vi "Demultiplexer_Laser80Simple160.vi"() -> ()   [LabVIEW 2012]
uses:
  <vilib>/Platform/TimedLoop/XDataNode/timing_clust.ctl
  <vilib>/Platform/TimedLoop/XDataNode/nitl_modes.ctl
  <vilib>/Platform/TimedLoop/XDataNode/wakeup.ctl
  <vilib>/rvi/Emulation/niFpgaSctlEmulationRegisterWithScheduler.vi
  <vilib>/rvi/eio/common/nirviEmuTemplateMethod_errors.vi
  <vilib>/rvi/Emulation/niFpgaSctlEmulationScheduler.vi
  <vilib>/rvi/FIFO/Fifo_Resource/nirvififoEmulationSetSize.vi
  <vilib>/rvi/DataTransferAndStorage/Container/Common/niFpgaContainerGetUniqueNameForEmu.vi
  <vilib>/rvi/errors/niFpgaSetErrorForExecOnDevCompSimple.vi
  <vilib>/rvi/eio/common/nirviEmuReportErrorAndStop.vi
  <vilib>/rvi/Emulation/niFpgaSctlEmulationFifoFullMgr.vi
  <vilib>/rvi/Emulation/niFpgaSctlEmulationResourceMgr.vi
  <vilib>/rvi/interface/RandomDataEmulation/nirviRandomDataFPGAFIFO.vi
  <vilib>/rvi/interface/RandomDataEmulation/niFpgaRandomDataHandleErrors.vi
  <vilib>/rvi/Emulation/niFpgaSctlEmulationGlobalWrite.vi
  <vilib>/Platform/TimedLoop/XDataNode/XDataNode.xnode
  <vilib>/eio/EIONode/EIONode.xnode
  <vilib>/rvi/DataTransferAndStorage/Container/XNode/niFpgaContainer.xnode
  <vilib>/rvi/FIFO/Fifo_Resource/nirvififoEmulationClear.vi
  <vilib>/rvi/FIFO/Fifo_Resource/nirvififoEmulationWrite.vi
  <vilib>/rvi/FIFO/Fifo_Resource/nirvififoEmulationRead.vi
  <vilib>/rvi/interface/RandomDataEmulation/nirviRandomDataFpgaReadWriteTemplate.vi
  <vilib>/Platform/TimedLoop/XDataNode/XDNodeRunTimeDep.lvlib
panel:
  out "Laser pulse count A1":u16
  out "ToHost FIFO Overflow A2Ch2":bool
  out "ToHost FIFO Overflow A2Ch1":bool
  out "ToHost FIFO Overflow A1Ch2":bool
  in  "Samples per pixel Acq A2":u16=10000 caption="Samples per pixel Acq"
  in  "Samples per pixel Acq A1":u16=10000 caption="Samples per pixel Acq"
  in  "Requested pixels A2":u32=100000 caption="Requested pixels"
  in  "Samples per pixel A2":u16=10000 caption="Samples per pixel"
  out "ToHost FIFO Overflow A1Ch1":bool
  out "Acquiring":bool
  in  "Wait for trigger":bool
  in  "Acquire continuously":bool=TRUE
  in  "Requested pixels A1":u32=100000 caption="Requested pixels"
  in  "Clear Interloop FIFO":bool
  out "Interloop FIFO overflow":bool
  in  "Samples per pixel A1":u16=10000 caption="Samples per pixel"
  in  "Acquire":bool
  out "Interloop FIFO timeout":bool
  in  "Commit":bool
  out "Xpoint_Switch_Ready":bool
  in  "Xpoint_Switch_Write":bool
  in  "Clock Source":u8(ring)=3 items=["Tristate"=0, "Sync Clock (PXIe only)"=2, "Adapter Module Onboard Clock"=3, "Strobe from Crosspoint Switch"=4, "Strobe Bypass"=5]
  in  "Onboard_Clock_Write":bool
  in  "Onboard_Clock_Write_Data":u16
  out "Onboard_Clock_Ready":bool
  in  "Acq_Reset":bool
  # "6587 IO module configuration"
  # "Demultiplexer - Laser 80MHzSimple160MHz"
  # "Acquisition control"
  # "Area 1"
  # "Area 2"
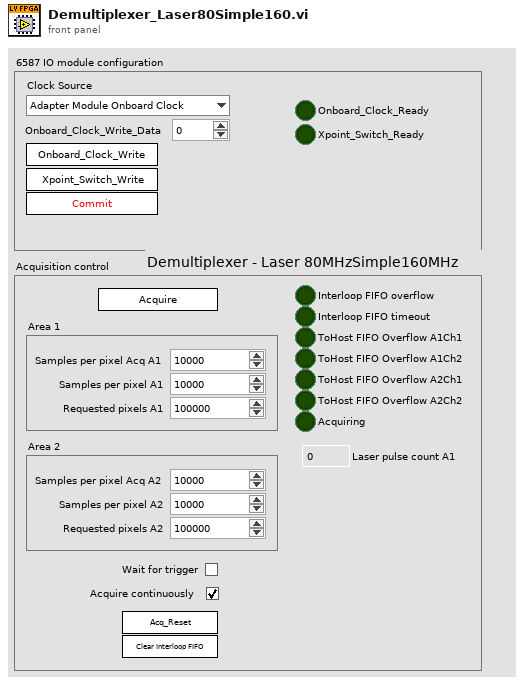
[diagram p1: front panel]
types:
  T1 = typedef "XDNodeRunTimeDep.lvlib/timing_clust.ctl" = cluster{"Expected End [f-1]":u64, "Actual End [f-1]":u64, "Finished Late? [f-1]":bool, "Expected End [i-1]":u64, "Actual End [i-1]":u64, "Finished Late? [i-1]":bool, "Expected Start [i]":u64, "Actual Start [i]":u64, "Expected Start [f]":u64, "Actual Start [f]":u64, "Source Name":string, "Structure Name":string, "Period":i64, "Deadline":i64, "Offset":i64, "Start":i64, "Priority":i32, "Timeout":i32, "Mode":T2, "Wakeup Reason":T3, "Error":errorcluster, "Source Type":string, "Secondary Source Type":string, "Global End Time":u64, "Global Start Time":u64, "Frame Duration":u64, "Iteration Duration":u64, "Assigned CPU":i32, "I/O Scan Engine Mode":u32}
  T2 = typedef "XDNodeRunTimeDep.lvlib/nitl_modes.ctl" = enum32{"No Change", "Process missed periods, maintain original phase", "Discard missed periods, maintain original phase", "Process missed periods, ignore original phase", "Discard missed periods, ignore original phase"}
  T3 = typedef "XDNodeRunTimeDep.lvlib/wakeup.ctl" = enum32{"Normal", "Aborted", "Asynchronous wakeup", "Timing source error", "Timed loop error", "Timeout"}
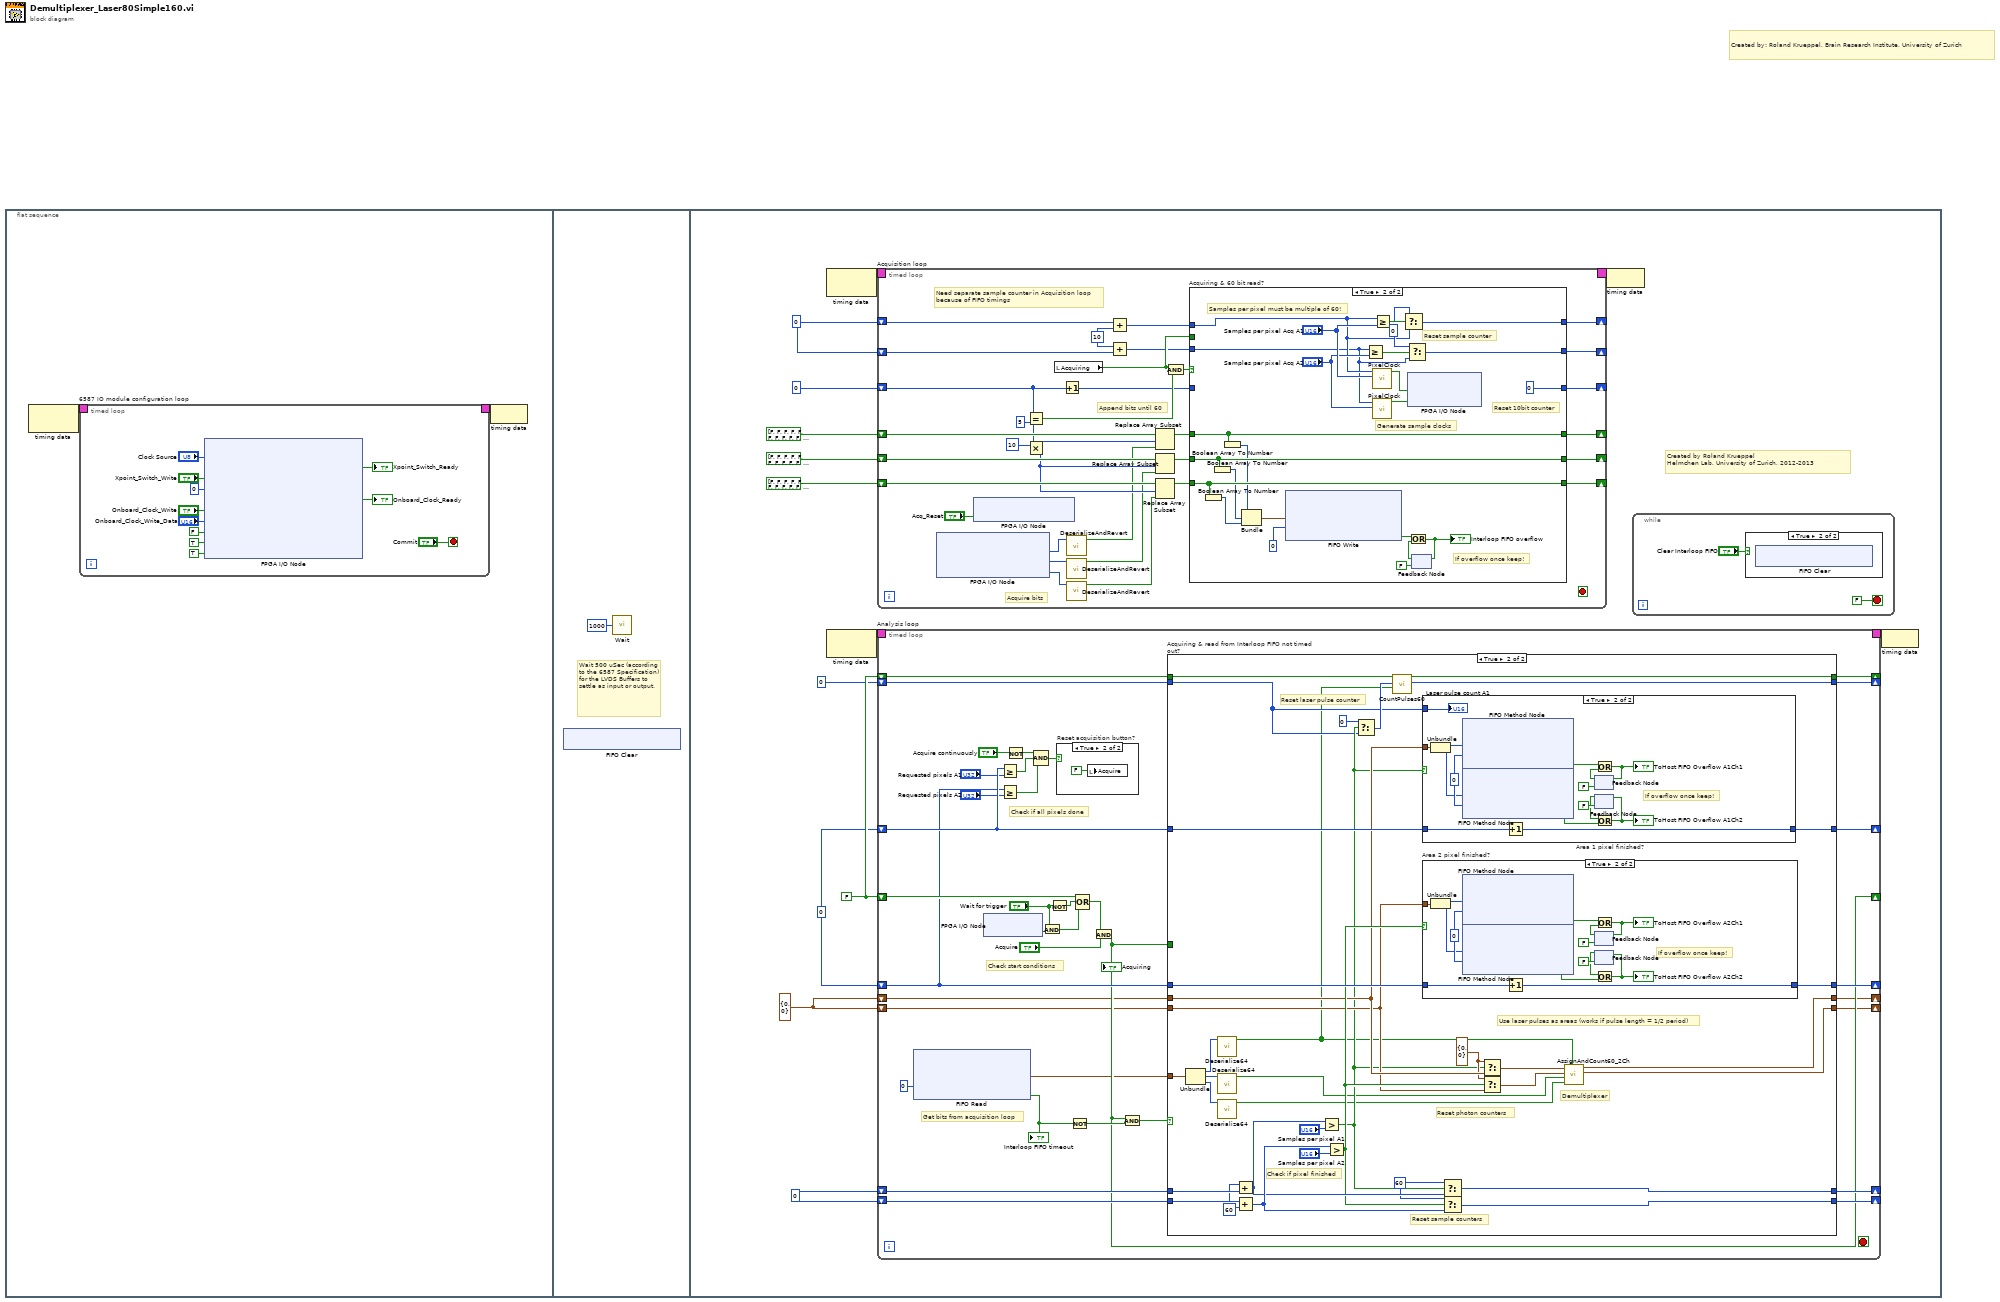
[diagram p0: block diagram]
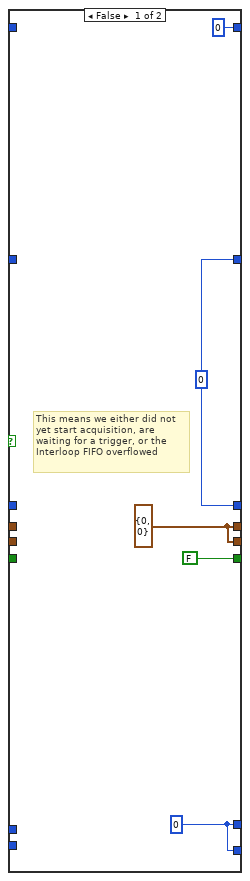
[diagram p5: hidden frame]
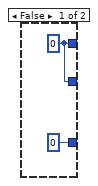
[diagram p9: hidden frame]
diagram:
  # "Created by: Roland Krueppel, Brain Research Institute, University of Zurich"
  n1 = flat-sequence {
    frame #0 {
      n2 = node-c288() -> (w2:T1)  [unwired: 1 in]
      n3 = timed-loop "6587 IO module configuration loop" {
        timing: w2 -> [_]
        timing-out: [_] -> w1
        stop <- "Commit" stop-if-true
        n4 = xnode "FPGA I/O Node"("IO Module\\Acq_IO_Clock_Source"="Clock Source", "IO Module\\Xpoint_Switch_Write"="Xpoint_Switch_Write", "IO Module\\LVDS_Data_Dir"=u16 0 ("IO Module\\LVDS_Data_Dir"), "IO Module\\Onboard_Clock_Write"="Onboard_Clock_Write", "IO Module\\Onboard_Clock_Write_Data"="Onboard_Clock_Write_Data", "IO Module\\SE_PFI0_WE"=FALSE ("IO Module\\SE_PFI0_WE"), "IO Module\\SE_PFI1_WE"=TRUE ("IO Module\\SE_PFI1_WE"), "IO Module\\SE_PFI2_WE"=TRUE ("IO Module\\SE_PFI2_WE")) -> ("IO Module\\Xpoint_Switch_Ready"=→"Xpoint_Switch_Ready":bool, "IO Module\\Onboard_Clock_Ready"=→"Onboard_Clock_Ready":bool)  [unwired: 10 in, 10 out]
      }
      n5 = node-c288(w1) -> ()
    }
    frame #1 {
      # "Wait 500 uSec (according to the 6587 Specification) for the LVDS Buffers to settle as input or output."
      n6 = xnode "FIFO Clear"() -> ()  [unwired: 1 in, 1 out]
      n7 = call "Wait"("Count(uSec)"=u32 1000) -> ()  [unwired: 1 out]
    }
    frame #2 {
      w21 = cluster{u16, u16} {0, 0} ("output cluster")
      w22 = u16 0
      w20 = u32 0 ("Cycle counter out")
      w23 = u16 0
      w24 = FALSE ("Last laser bit out")
      # "Created by Roland Krueppel\nHelmchen Lab, University of Zurich, 2012-2013"
      n8 = node-c288() -> (w32:T1)  [unwired: 1 in]
      n9 = node-c288() -> (w30:T1)  [unwired: 1 in]
      n10 = timed-loop "Acquisition loop" {
        timing: w32 -> [_]
        timing-out: [_] -> w31
        shift-right: [w195] -> _
        shift-left: bool[] [FALSE, FALSE, FALSE, FALSE, FALSE, FALSE, FALSE, FALSE, FALSE, FALSE, FALSE, FALSE, FALSE, FALSE, FALSE, FALSE, FALSE, FALSE, FALSE, FALSE, FALSE, FALSE, FALSE, FALSE, FALSE, FALSE, FALSE, FALSE, FALSE, FALSE, FALSE, FALSE, FALSE, FALSE, FALSE, FALSE, FALSE, FALSE, FALSE, FALSE, FALSE, FALSE, FALSE, FALSE, FALSE, FALSE, FALSE, FALSE, FALSE, FALSE, FALSE, FALSE, FALSE, FALSE, FALSE, FALSE, FALSE, FALSE, FALSE, FALSE, FALSE, FALSE, FALSE, FALSE] ("Boolean array") -> [w203]
        shift-right: [w194] -> _
        shift-left: bool[] [FALSE, FALSE, FALSE, FALSE, FALSE, FALSE, FALSE, FALSE, FALSE, FALSE, FALSE, FALSE, FALSE, FALSE, FALSE, FALSE, FALSE, FALSE, FALSE, FALSE, FALSE, FALSE, FALSE, FALSE, FALSE, FALSE, FALSE, FALSE, FALSE, FALSE, FALSE, FALSE, FALSE, FALSE, FALSE, FALSE, FALSE, FALSE, FALSE, FALSE, FALSE, FALSE, FALSE, FALSE, FALSE, FALSE, FALSE, FALSE, FALSE, FALSE, FALSE, FALSE, FALSE, FALSE, FALSE, FALSE, FALSE, FALSE, FALSE, FALSE, FALSE, FALSE, FALSE, FALSE] ("Boolean array") -> [w202]
        shift-right: [w193] -> _
        shift-left: 0 -> [w192]
        shift-right: [w188] -> _
        shift-left: bool[] [FALSE, FALSE, FALSE, FALSE, FALSE, FALSE, FALSE, FALSE, FALSE, FALSE, FALSE, FALSE, FALSE, FALSE, FALSE, FALSE, FALSE, FALSE, FALSE, FALSE, FALSE, FALSE, FALSE, FALSE, FALSE, FALSE, FALSE, FALSE, FALSE, FALSE, FALSE, FALSE, FALSE, FALSE, FALSE, FALSE, FALSE, FALSE, FALSE, FALSE, FALSE, FALSE, FALSE, FALSE, FALSE, FALSE, FALSE, FALSE, FALSE, FALSE, FALSE, FALSE, FALSE, FALSE, FALSE, FALSE, FALSE, FALSE, FALSE, FALSE, FALSE, FALSE, FALSE, FALSE] ("Boolean array") -> [w191]
        shift-right: [w187] -> _
        shift-left: w22 -> [w177]
        shift-right: [w186] -> _
        shift-left: w22 -> [w175]
        stop <- _ stop-if-true
        w173 = u16 10 ("y")
        # "Need separate sample counter in Acquisition loop\nbecause of FIFO timings"
        # "Append bits until 60"
        # "Acquire bits"
        n11 = xnode "FPGA I/O Node"() -> ("IO Module\\LVDS_Ch0_Rd"=w183:u16, "IO Module\\LVDS_Ch1_Rd"=w181:u16, "IO Module\\LVDS_Ch2_Rd"=w179:u16)  [unwired: 3 in, 3 out]
        n12 = xnode "FPGA I/O Node"("IO Module\\Acq_Reset"="Acq_Reset") -> ()  [unwired: 1 in, 1 out]
        n13 = Equal?(x=w192, y=5) -> (x = y?=w199:bool)
        n14 = Multiply(x=10 ("y"), y=w192) -> (x*y=w190:i32)
        n15 = local read "Acquiring"() -> (w185:bool)
        n16 = Increment(x=w192) -> (x+1=w184:i32)
        n17 = call "DeserializeAndRevert.vi"("U16 input"=w183) -> ("10bit output"=w182:bool[])  [unwired: 10 in]
        n18 = call "DeserializeAndRevert.vi"("U16 input"=w181) -> ("10bit output"=w180:bool[])  [unwired: 10 in]
        n19 = call "DeserializeAndRevert.vi"("U16 input"=w179) -> ("10bit output"=w178:bool[])  [unwired: 10 in]
        n20 = Add(x=w177, y=w173) -> (x+y=w176:u16)
        n21 = Add(x=w173, y=w175) -> (x+y=w174:u16)
        n22 = Replace Array Subset(array=w203, new element=w182, index=w190) -> (w197:bool[])
        n23 = Replace Array Subset(array=w202, new element=w180, index=w190) -> (w196:bool[])
        n24 = Replace Array Subset(array=w191, new element=w178, index=w190) -> (w189:bool[])
        n25 = And(x=w185, y=w199) -> (x .and. y?=w198:bool)
        n26 = case "Acquiring & 60 bit read?" shown="True" w198 {
          tunnel: w197 -> [w214 w240]
          tunnel: w196 -> [w213 w242]
          tunnel: [w214 w240] -> w195
          tunnel: [w213 w242] -> w194
          tunnel: [w205 0] -> w193
          tunnel: w184 -> [w206 _]
          tunnel: w189 -> [w212 w241]
          tunnel: [w212 w241] -> w188
          tunnel: w176 -> [w210 w225]
          tunnel: [w207 w238] -> w187
          tunnel: w174 -> [w209 w224]
          tunnel: [w208 w233] -> w186
          tunnel: w185 -> [w211 _]
          frame False {
            n27 = case "Acquiring?" shown="True" w211 {
              tunnel: w210 -> [_ w219]
              tunnel: w209 -> [_ w218]
              tunnel: [w216 w219] -> w207
              tunnel: [w216 w218] -> w208
              tunnel: w206 -> [_ w217]
              tunnel: [0 w217] -> w205
              frame False {
                w216 = u16 0
              }
              frame True {
              }
            }
          }
          frame True {
            w234 = u16 0 ("t")
            # "Reset 10bit counter"
            # "Samples per pixel must be multiple of 60!"
            # "Reset sample counter"
            # "If overflow once keep!"
            # "Generate sample clocks"
            n28 = Boolean Array To Number(Boolean array=w241) -> (number=w228:u64)
            n29 = Boolean Array To Number(Boolean array=w242) -> (number=w229:u64)
            n30 = Boolean Array To Number(Boolean array=w240) -> (number=w230:u64)
            n31 = Bundle(w230, w229, w228) -> (w227:cluster{u64, u64, u64})  [unwired: 1 in]
            n32 = xnode ("FIFO Write")("Element"=w227, "Timeout"=0) -> ("Timed Out?"=w223:bool)  [unwired: 1 in, 1 out]
            n33 = Greater Or Equal?(x=w224, y="Samples per pixel Acq A2") -> (x >= y?=w235:bool)
            n34 = call "PixelClock.vi"("Samples per pixel"="Samples per pixel Acq A1", "Sample counter"=w225) -> ("Pixel clock"=w236:bool)  [unwired: 9 in]
            n35 = call "PixelClock.vi"("Samples per pixel"="Samples per pixel Acq A2", "Sample counter"=w224) -> ("Pixel clock"=w231:bool)  [unwired: 9 in]
            n36 = Greater Or Equal?(x=w225, y="Samples per pixel Acq A1") -> (x >= y?=w239:bool)
            n37 = Select(t=w234, s=w239, f=w225) -> (s? t:f=w238:u16)
            n38 = Select(t=w234, s=w235, f=w224) -> (s? t:f=w233:u16)
            n39 = xnode "FPGA I/O Node"("Pixel clock A1"=w236, "Pixel clock A2"=w231) -> ()  [unwired: 2 in, 2 out]
            n40 = feedback #1(FALSE) -> (w221:bool)
            n41 = Or(x=w223, y=w221) -> (x .or. y?=w222:bool)
            "Interloop FIFO overflow" <- w222
            n42 = feedback-in #1(w222) -> ()
          }
        }
      }
      n43 = timed-loop "Analysis loop" {
        timing: w30 -> [_]
        timing-out: [_] -> w29
        shift-right: [w70] -> _
        shift-left: w24 -> [w69]
        shift-right: [w48] -> _
        shift-left: w23 -> [w68]
        shift-right: [w46] -> _
        shift-left: w20 -> [w67]
        shift-right: [w44] -> _
        shift-left: w24 -> [w56]
        shift-right: [w47] -> _
        shift-left: w23 -> [w54]
        shift-right: [w45] -> _
        shift-left: w20 -> [w52]
        shift-right: [w39] -> _
        shift-left: w21 -> [w41]
        shift-right: [w38] -> _
        shift-left: w21 -> [w40]
        shift-right: [w37] -> _
        shift-left: u16 0 ("New pulse count") -> [w36]
        stop <- _ stop-if-true
        # "Get bits from acquisition loop"
        # "Check start conditions"
        # "Check if all pixels done"
        n44 = xnode ("FIFO Read")("Timeout"=0) -> ("Element"=w35:cluster{"Laser":u64, "Ch0":u64, "Ch1":u64}, "Timed Out?"=w42:bool)  [unwired: 1 in, 1 out]
        "Interloop FIFO timeout" <- w42
        n45 = xnode "FPGA I/O Node"() -> ("TriggerIn"=w62:bool)  [unwired: 1 in, 1 out]
        n46 = Greater Or Equal?(x=w67, y="Requested pixels A1") -> (x >= y?=w50:bool)
        n47 = Greater Or Equal?(x=w52, y="Requested pixels A2") -> (x >= y?=w49:bool)
        n48 = Not(x="Acquire continuously") -> (.not. x?=w51:bool)
        n49 = Compound Arithmetic op=AND(w51, w50, w49) -> (w64:bool)
        n50 = And(x="Wait for trigger", y=w62) -> (x .and. y?=w59:bool)
        n51 = Not(x="Wait for trigger") -> (.not. x?=w60:bool)
        n52 = case "Reset acquisition button?" shown="True" w64 {
          frame False {
          }
          frame True {
            n53 = local write "Acquire"(FALSE ("Acquire")) -> ()
          }
        }
        n54 = Not(x=w42) -> (.not. x?=w57:bool)
        n55 = Compound Arithmetic op=OR(w56, w60, w59) -> (w58:bool)
        n56 = And(x=w58, y="Acquire") -> (x .and. y?=w44:bool)
        "Acquiring" <- w44
        n57 = And(x=w44, y=w57) -> (x .and. y?=w55:bool)
        n58 = case "Acquiring & read from Interloop FIFO not timed out?" shown="True" w55 {
          tunnel: w41 -> [w87 w122]
          tunnel: [w83 w102] -> w70
          tunnel: w69 -> [w84 w111]
          tunnel: w68 -> [w86 w137]
          tunnel: w67 -> [w85 w133]
          tunnel: w44 -> [w88 _]
          tunnel: w54 -> [w77 w135]
          tunnel: w52 -> [w80 w132]
          tunnel: [w78 w125] -> w48
          tunnel: [w76 w127] -> w47
          tunnel: [w82 w117] -> w39
          tunnel: [w81 w130] -> w46
          tunnel: [w79 w131] -> w45
          tunnel: w40 -> [w75 w120]
          tunnel: [w74 w116] -> w38
          tunnel: [w72 w115] -> w37
          tunnel: w36 -> [w73 w110]
          tunnel: w35 -> [_ w106]
          frame False {
            n59 = case "Acquiring?" shown="True" w88 {
              tunnel: w87 -> [_ w100]
              tunnel: w86 -> [_ w97]
              tunnel: w85 -> [_ w99]
              tunnel: w84 -> [_ w101]
              tunnel: [FALSE ("Last laser bit out") w101] -> w83
              tunnel: [w91 w100] -> w82
              tunnel: [w92 w99] -> w81
              tunnel: w80 -> [_ w98]
              tunnel: [w92 w98] -> w79
              tunnel: [w90 w97] -> w78
              tunnel: [w90 w96] -> w76
              tunnel: w77 -> [_ w96]
              tunnel: w75 -> [_ w95]
              tunnel: [w91 w95] -> w74
              tunnel: w73 -> [_ w94]
              tunnel: [u16 0 ("New pulse count") w94] -> w72
              frame False {
                w91 = cluster{u16, u16} {0, 0} ("output cluster")
                w92 = u32 0 ("Cycle counter out")
                w90 = u16 0
                # "This means we either did not\nyet start acquisition, are\nwaiting for a trigger, or the\nInterloop FIFO overflowed"
              }
              frame True {
                # "This means we are\nreading faster here\nthan acquiring in\nAcquisition loop\n-> keep all values"
              }
            }
          }
          frame True {
            w118 = cluster{u16, u16} {0, 0} ("t")
            w124 = u16 60 ("t")
            w134 = u16 60
            # "Reset laser pulse counter"
            # "Demultiplexer"
            # "Reset photon counters"
            # "Use laser pulses as areas (works if pulse length = 1/2 period)"
            # "Check if pixel finished"
            # "Reset sample counters"
            n60 = Unbundle(w106) -> ("Laser"=w107:u64, "Ch0"=w108:u64, "Ch1"=w109:u64)
            n61 = call "Deserialize64.vi"("U64 input"=w107) -> ("60bit output"=w105:bool[])  [unwired: 10 in]
            n62 = call "Deserialize64.vi"("U64 input"=w108) -> ("60bit output"=w104:bool[])  [unwired: 10 in]
            n63 = call "Deserialize64.vi"("U64 input"=w109) -> ("60bit output"=w103:bool[])  [unwired: 10 in]
            n64 = Add(x=w134, y=w137) -> (x+y=w126:u16)
            n65 = Add(x=w135, y=w134) -> (x+y=w128:u16)
            n66 = Greater?(x=w126, y="Samples per pixel A1") -> (0:w114:bool)
            n67 = Greater?(x=w128, y="Samples per pixel A2") -> (0:w123:bool)
            n68 = Select(t=u16 0, s=w114, f=w110) -> (s? t:f=w113:u16)
            n69 = call "CountPulses60.vi"("60bit input"=w105, "Previous pulse count"=w113, "Last sample"=w111) -> ("New pulse count"=w115:u16, "New last sample"=w102:bool)  [unwired: 7 in]
            n70 = case "Area 1 pixel finished?" shown="True" w114 {
              tunnel: w122 -> [_ w165]
              tunnel: w133 -> [w153 w167]
              tunnel: [w153 w166] -> w130
              tunnel: w110 -> [_ w162]
              frame False {
              }
              frame True {
                w168 = 0 ("Timeout")
                # "If overflow once keep!"
                n71 = Unbundle(w165) -> (w164:u16, w163:u16)
                n72 = xnode ("FIFO Method Node")("Element"=w164, "Timeout"=w168) -> ("Timed Out?"=w157:bool)  [unwired: 1 in, 1 out]
                n73 = xnode ("FIFO Method Node")("Element"=w163, "Timeout"=w168) -> ("Timed Out?"=w156:bool)  [unwired: 1 in, 1 out]
                n74 = Increment(x=w167) -> (x+1=w166:u32)
                n75 = feedback #2(FALSE) -> (w161:bool)
                n76 = feedback #3(FALSE) -> (w158:bool)
                n77 = Or(x=w157, y=w161) -> (x .or. y?=w155:bool)
                "ToHost FIFO Overflow A1Ch1" <- w155
                n78 = feedback-in #2(w155) -> ()
                n79 = Or(x=w158, y=w156) -> (x .or. y?=w154:bool)
                "ToHost FIFO Overflow A1Ch2" <- w154
                n80 = feedback-in #3(w154) -> ()
                "Laser pulse count A1" <- w162
              }
            }
            n81 = case "Area 2 pixel finished?" shown="True" w123 {
              tunnel: w132 -> [w138 w151]
              tunnel: [w138 w150] -> w131
              tunnel: w120 -> [_ w149]
              frame False {
              }
              frame True {
                w152 = 0 ("Timeout")
                # "If overflow once keep!"
                n82 = Unbundle(w149) -> (w148:u16, w147:u16)
                n83 = xnode ("FIFO Method Node")("Element"=w148, "Timeout"=w152) -> ("Timed Out?"=w142:bool)  [unwired: 1 in, 1 out]
                n84 = xnode ("FIFO Method Node")("Element"=w147, "Timeout"=w152) -> ("Timed Out?"=w141:bool)  [unwired: 1 in, 1 out]
                n85 = Increment(x=w151) -> (x+1=w150:u32)
                n86 = feedback #4(FALSE) -> (w146:bool)
                n87 = feedback #5(FALSE) -> (w143:bool)
                n88 = Or(x=w142, y=w146) -> (x .or. y?=w140:bool)
                "ToHost FIFO Overflow A2Ch1" <- w140
                n89 = feedback-in #4(w140) -> ()
                n90 = Or(x=w143, y=w141) -> (x .or. y?=w139:bool)
                "ToHost FIFO Overflow A2Ch2" <- w139
                n91 = feedback-in #5(w139) -> ()
              }
            }
            n92 = Select(t=w124, s=w114, f=w126) -> (s? t:f=w125:u16)
            n93 = Select(t=w124, s=w123, f=w128) -> (s? t:f=w127:u16)
            n94 = Select(t=w118, s=w114, f=w122) -> (s? t:f=w121:cluster{u16, u16})
            n95 = Select(t=w118, s=w123, f=w120) -> (s? t:f=w119:cluster{u16, u16})
            n96 = call "AssignAndCount60_2Ch.vi"("Area bits in"=w105, "PMT bits Ch2 in"=w103, "PMT bits Ch1 in"=w104, "Photon counters area 2 in"=w119, "Photon counters area 1 in"=w121) -> ("Photon counters area 2 out"=w116:cluster{u16, u16}, "Photon counters area 1 out"=w117:cluster{u16, u16})  [unwired: 5 in]
          }
        }
      }
      n97 = node-c288(w31) -> ()
      n98 = while {
        stop <- FALSE stop-if-true
        n99 = case shown="True" "Clear Interloop FIFO" {
          frame False {
          }
          frame True {
            n100 = xnode ("FIFO Clear")() -> ()  [unwired: 1 in, 1 out]
          }
        }
      }
      n101 = node-c288(w29) -> ()
    }
  }
